vi "Set IP.vi"(8 "error in (no error)":errorcluster, 9 "IP":string, 10 "ID":string, 11 "Guardian List in":refnum<class "Guardian List.lvclass">) -> (0 "error out":errorcluster, 3 "Guardian List out":refnum<class "Guardian List.lvclass">)   [LabVIEW 2026, in "TALOS.lvlib" / "Classes.lvlib" / "Guardian List.lvclass"]
uses:
  Guardian List.lvclass
  Guardian List.lvclass/Guardian List.ctl
  Ancestor/Ancestor/Ancestor.lvclass/Ancestor.ctl
  FGV/Error Memory/Get Error Description.vi
  Support VIs/Get PC name.vi
  Ancestor/Ancestor/Read ID.vi
  Support VIs/Get Class Name.vi
  <vilib>/Utility/error.llb/Clear Errors.vi
  FGV/Error Memory/Error Memory Core.vi
  <vilib>/AdvancedString/Delimited String to 1D String Array.vi
  <vilib>/AdvancedString/Delimited String to 1D String Array (string).vi
  Support VIs/Circus Root Path.vi
  FGV/Error Memory/Error Crt Lvl checker.vi
  FGV/Error Memory/Error Memory Core.vi/40c8088d-b597-4017-91af-faa98e00292e.vi
  FGV/Error Memory/Error Memory Core.vi/d4a3ab98-063c-4e44-b43d-fbdcfe6c2be2.vi
  Support VIs/Global Memory.vi
  <vilib>/Utility/LVClass/Get LV Class Name.vi
  Support VIs/Is in Packed Library.vi
  Support VIs/TALOS Root path.vi
  Support VIs/Read CSV worksheet.vi
  Support VIs/Global Constants.vi
  <vilib>/Utility/error.llb/General Error Handler.vi
  Ancestor/Ancestor/Ancestor.lvclass
  <vilib>/Comparison/Equal/Equal Functor/Equal Functor.lvclass
  TALOS.lvlib
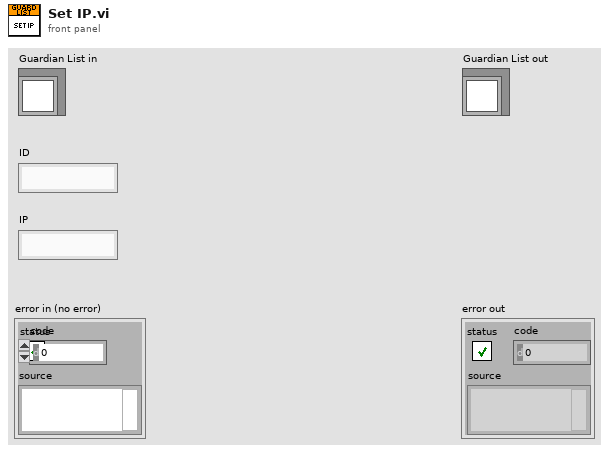
[diagram p1: front panel]
types:
  T1 = typedef "TALOS.lvlib/Classes.lvlib/Guardian List.lvclass/Guardian Properties.ctl" = cluster{"Alive":bool, "Last Seen":timestamp, "IP":string, "TCP Writer associated ID":string, "uS List received":bool, "Abort":bool, "Bearer":bool, "TCP Listener associated ID":string}
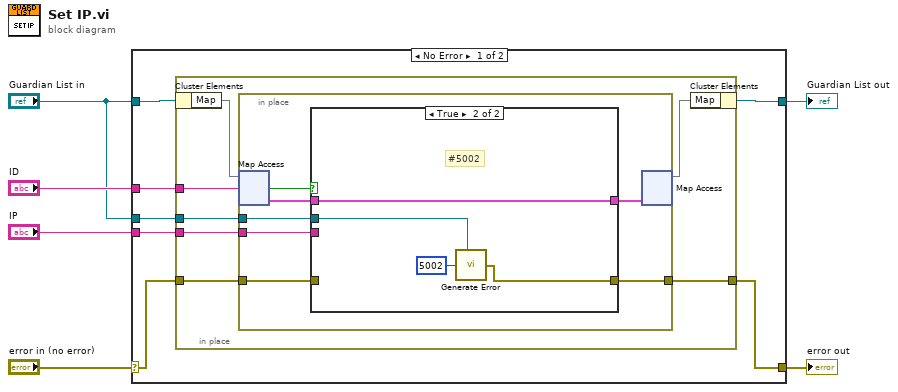
[diagram p0: block diagram]
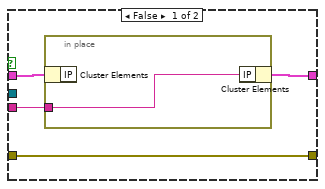
[diagram p2: hidden frame]
diagram:
  n1 = case shown="No Error" "error in (no error)" {
    selector: "error in (no error)" -> [w8 w38]
    tunnel: [w7 w38] -> w5
    tunnel: [w11 w37] -> w4
    tunnel: "Guardian List in" -> [w12 w37]
    tunnel: "ID" -> [w13 _]
    tunnel: "IP" -> [w10 _]
    tunnel: "Guardian List in" -> [w9 _]
    frame No Error {
      n2 = in-place {
        in-place-border: w13 -> [w20]
        in-place-border: w10 -> [w17]
        in-place-border: w9 -> [w16]
        in-place-border: w8 -> [w15]
        in-place-border: [w14] -> w7
        n3 = in-place-cluster #1(w12) -> ("Map"=w19:map{string, T1})
        n4 = in-place {
          in-place-border: w17 -> [w25]
          in-place-border: w16 -> [w21]
          in-place-border: w15 -> [w23]
          in-place-border: [w22] -> w14
          n5 = in-place-map #2(w19, w20) -> (w27:T1, w24:bool)  [unwired: 1 in]
          n6 = case shown="True" w24 {
            tunnel: w27 -> [w31 w36]
            tunnel: [w30 w36] -> w26
            tunnel: w25 -> [w29 _]
            tunnel: w23 -> [w28 _]
            tunnel: [w28 w35] -> w22
            tunnel: w21 -> [_ w34]
            frame False {
              n7 = in-place {
                in-place-border: w29 -> [w32]
                n8 = in-place-cluster #3(w31) -> ()  [unwired: 1 out]
                n9 = in-place-cluster #3("IP"=w32) -> (w30:T1)
              }
            }
            frame True {
              # "#5002"
              n10 = call "Generate Error.vi"("Class"=w34, "Error Code"=5002) -> ("error out"=w35:errorcluster)  [unwired: 5 in]
            }
          }
          n11 = in-place-map #2(w26) -> (w18:map{string, T1})  [unwired: 1 in, 2 out]
        }
        n12 = in-place-cluster #1("Map"=w18) -> (w11:refnum<class "Guardian List.lvclass">)
      }
    }
    frame Error {
    }
  }
  "error out" <- w5
  "Guardian List out" <- w4
